vi "Disabled controls when rec. (FGV) .vi"(8 "error in (no error)":errorcluster, 10 "Enum":enum16{"Read", "Write"}(ring), 11 "Array of controls":refnum<vi>[](array[refnum])) -> (0 "error out":errorcluster, 3 "Array of controls":refnum<vi>[](array[refnum]))   [LabVIEW 2014]
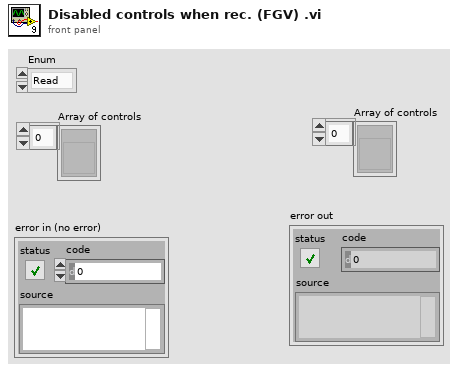
[diagram p1: front panel]
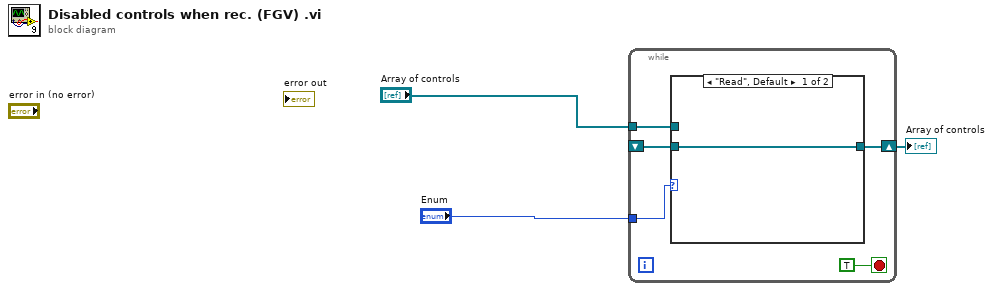
[diagram p0: block diagram]
diagram:
  n1 = while {
    tunnel: "Enum" -> [w7]
    shift-right: [w6] -> w1
    shift-left: _ -> [w4]
    tunnel: "Array of controls" -> [w5]
    stop <- TRUE stop-if-true
    n2 = case shown="\"Read\", Default" w7 {
      tunnel: [w9 w10] -> w6
      tunnel: w5 -> [_ w10]
      tunnel: w4 -> [w9 _]
      frame "Read", Default {
      }
      frame "Write" {
      }
    }
  }
  "Array of controls" <- w1
